vi "SetPressure_v2.vi"(2 "Debug Mode":bool, 3 "Elapsed Time (s)":dbl, 4 "State":enum16{"Edit", "Start", "Run", "End", "Idle"}(ring), 5 "Argument List In":string[](array[string])) -> (0 "Status Out":string, 1 "Argument List Out":string[](array[string]))   [LabVIEW 2011]
panel:
  out "error out":errorcluster
  in  "Dilution factor":dbl min=0.0 max=10.0 format="%.2f"
  in  "Set Point":string(combo)="C"
  in  "P (Torr)":dbl=20.0 format="%.1f"
  in  "Cancel":bool
  in  "OK":bool
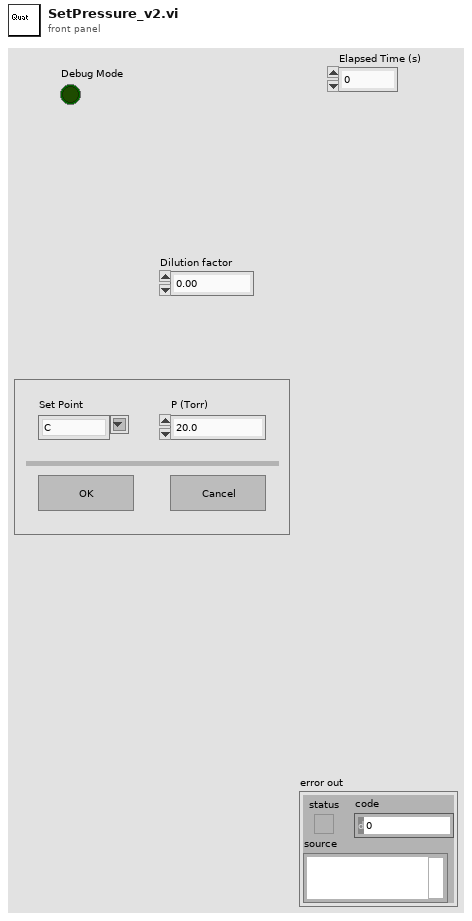
[diagram p1: front panel]
types:
  T1 = enum16{"Discrete", "Continuous", "Instantaneous"}
  T2 = enum32{"Invalid", "Default", "Floating", "Floating/Auto-Hide", "Modal"}
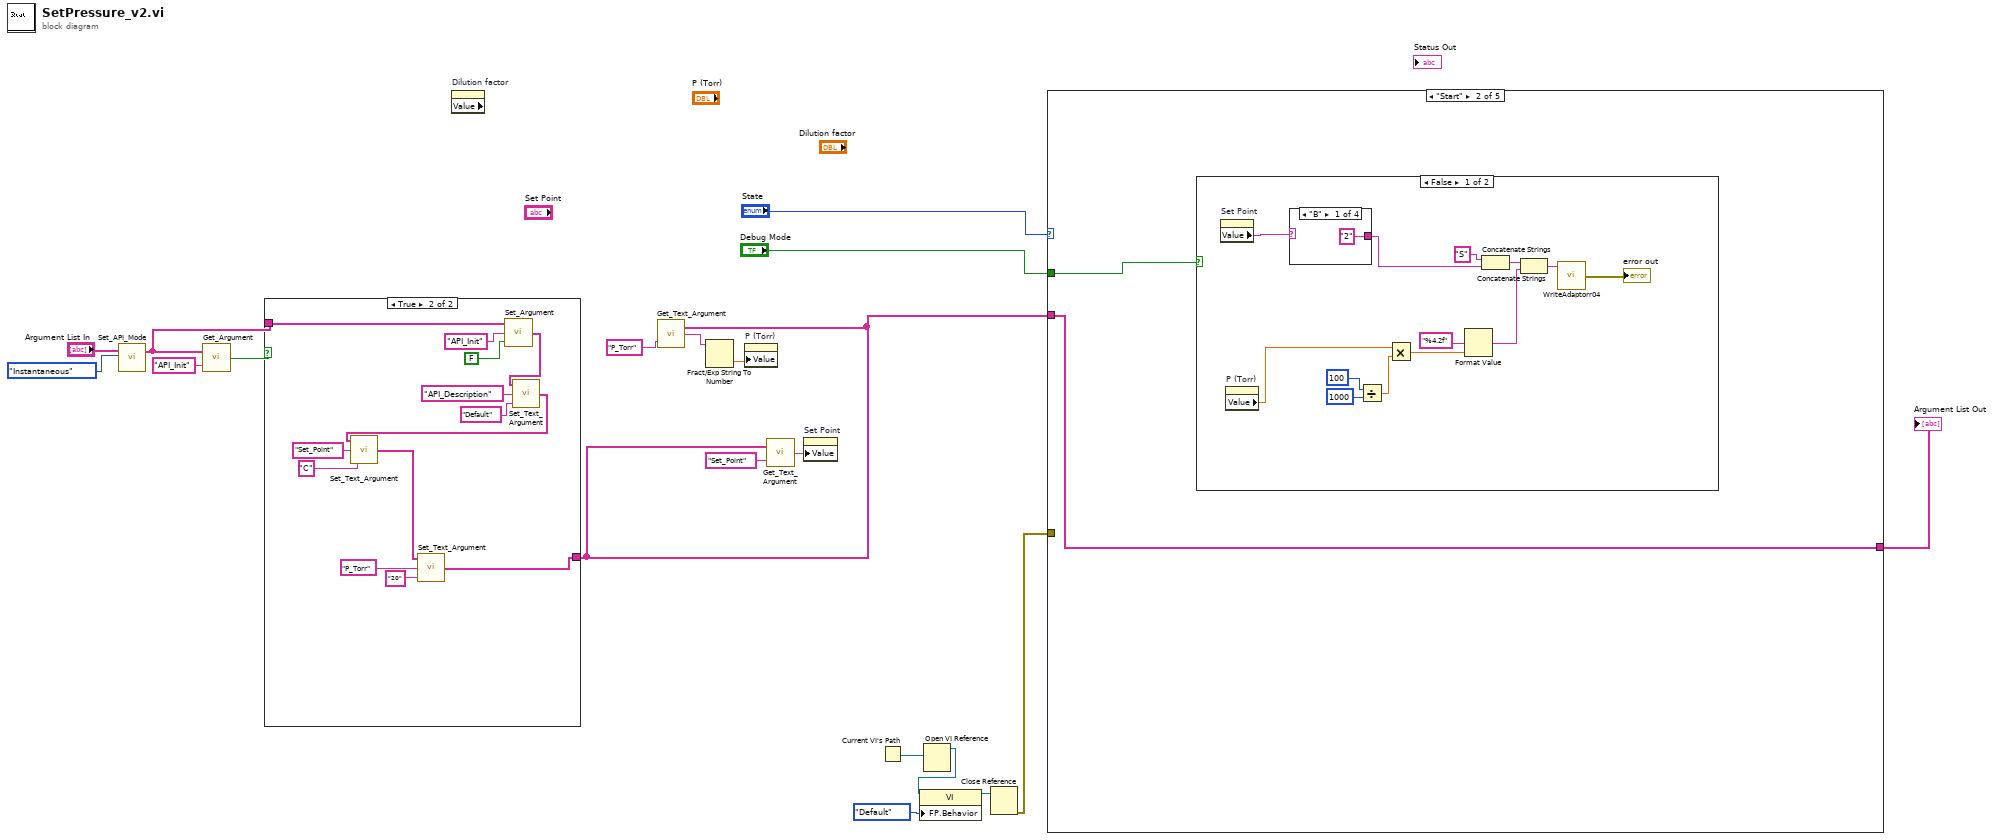
[diagram p0: block diagram]
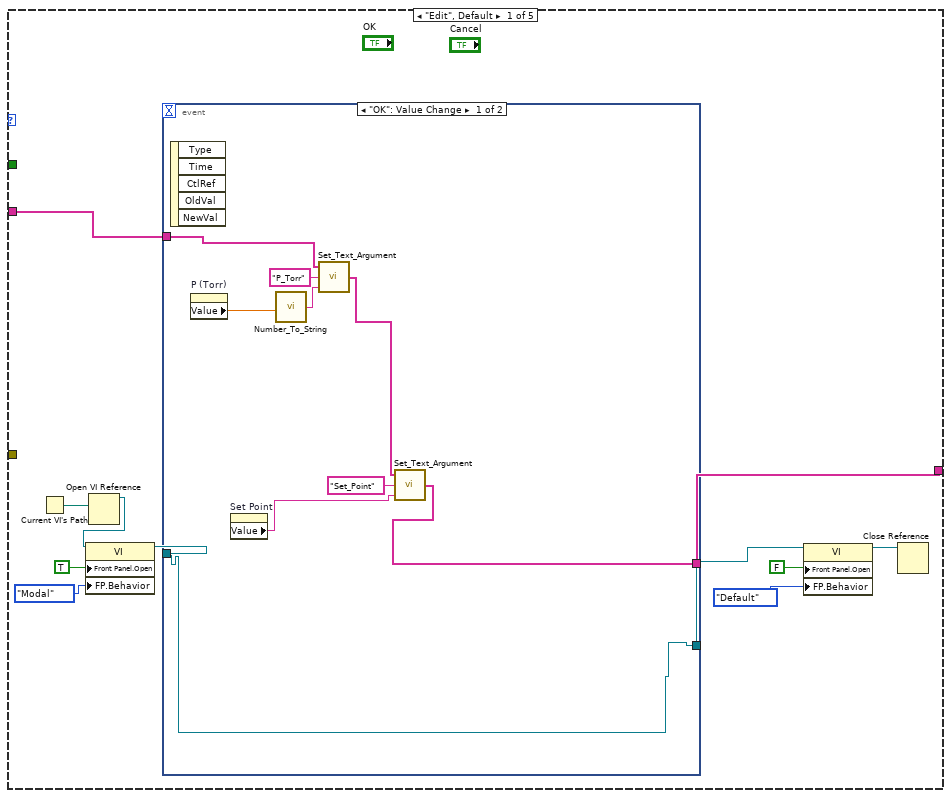
[diagram p3: hidden frame]
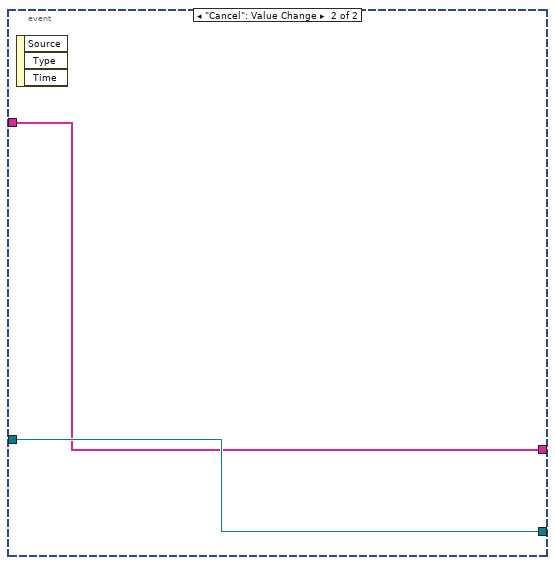
[diagram p4: hidden frame]
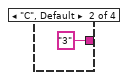
[diagram p5: hidden frame]
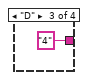
[diagram p6: hidden frame]
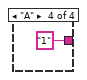
[diagram p7: hidden frame]
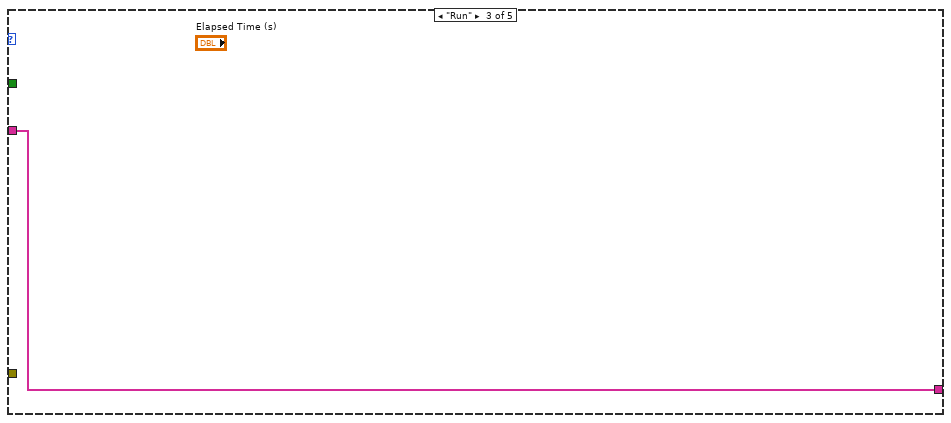
[diagram p9: hidden frame]
diagram:
  n1 = call "Set_API_Mode.vi"("API Mode"=T1."Instantaneous", "Argument List In"="Argument List In") -> ("Argument List Out"=w7:string[])  [unwired: 3 in]
  n2 = call "Get_Argument.vi"("Argument"="API_Init", "Argument List"=w7) -> ("Enabled"=w8:bool)
  n3 = case shown="True" w8 {
    tunnel: w7 -> [w20 w33]
    tunnel: [w20 w23] -> w3
    frame False {
    }
    frame True {
      n4 = call "Set_Argument.vi"("Enable"=FALSE, "Argument"="API_Init", "Argument List In"=w33) -> ("Argument List Out"=w30:string[])
      n5 = call "Set_Text_Argument.vi"("Text"="Default", "Argument"="API_Description", "Argument List In"=w30) -> ("Argument List Out"=w25:string[])
      n6 = call "Set_Text_Argument.vi"("Text"="C", "Argument"="Set_Point", "Argument List In"=w25) -> ("Argument List Out"=w24:string[])
      n7 = call "Set_Text_Argument.vi"("Text"="20", "Argument"="P_Torr", "Argument List In"=w24) -> ("Argument List Out"=w23:string[])
    }
  }
  n8 = property on="Dilution factor" class="DigNum (strict)" props=["Value"]() -> ()  [unwired: 2 in, 3 out]
  n9 = call "Get_Text_Argument.vi"("Argument"="P_Torr", "Argument List"=w3) -> ("Text"=w5:string)
  n10 = Fract/Exp String To Number(string=w5) -> (number=w4:dbl)  [unwired: 4 out]
  n11 = property on="P (Torr)" class="DigNum (strict)"("Value"=w4) -> ()  [unwired: 2 in, 2 out]
  n12 = call "Get_Text_Argument.vi"("Argument"="Set_Point", "Argument List"=w3) -> ("Text"=w1:string)
  n13 = property on="Set Point" class="CmbBox"("Value"=w1) -> ()  [unwired: 2 in, 2 out]
  n14 = Current VI's Path() -> (path=w16:path)
  n15 = Open VI Reference(vi path=w16) -> (vi reference=w15:refnum<vi>)  [unwired: 1 in, 5 out]
  n16 = property class="VI"(reference=w15, "FP.Behavior"=T2."Default" ("Front Panel Window:Behavior")) -> (reference out=w13:refnum<vi>)  [unwired: 1 in, 1 out]
  n17 = Close Reference(reference=w13) -> (error out=w12:errorcluster)  [unwired: 1 in]
  n18 = case shown="\"Start\"" "State" {
    tunnel: [w44 w57 w75 w76 w77] -> w18
    tunnel: w3 -> [w43 w57 w75 w76 w77]
    tunnel: "Debug Mode" -> [_ w56 _ _ _]
    tunnel: w12 -> [_ _ _ _ _]
    frame "Edit", Default {
      n19 = Current VI's Path() -> (path=w38:path)
      n20 = Open VI Reference(vi path=w38) -> (vi reference=w37:refnum<vi>)  [unwired: 1 in, 5 out]
      n21 = property class="VI"(reference=w37, "Front Panel.Open"=TRUE ("Front Panel Window:Open"), "FP.Behavior"=T2."Modal" ("Front Panel Window:Behavior")) -> (reference out=w41:refnum<vi>)  [unwired: 1 in, 1 out]
      n22 = event shown="[0] \"OK\": Value Change" {
        selector: _ -> [_ _]
        dyn-events: _ -> [_ _]
        timeout: _ -> [_ _]
        tunnel: w43 -> [w50 w54]
        tunnel: [w46 w54] -> w44
        tunnel: [w48 w55] -> w40
        tunnel: w41 -> [w48 w55]
        event "OK": Value Change {
          n23 = event-data() -> ()  [unwired: 6 out]
          n24 = property on="P (Torr)" class="DigNum (strict)"() -> ("Value"=w47:dbl)  [unwired: 2 in, 2 out]
          n25 = property on="Set Point" class="CmbBox"() -> ("Value"=w45:string)  [unwired: 2 in, 2 out]
          n26 = call "Number_To_String.vi"("Number"=w47) -> ("String"=w51:string)
          n27 = call "Set_Text_Argument.vi"("Text"=w51, "Argument"="P_Torr", "Argument List In"=w50) -> ("Argument List Out"=w49:string[])
          n28 = call "Set_Text_Argument.vi"("Text"=w45, "Argument"="Set_Point", "Argument List In"=w49) -> ("Argument List Out"=w46:string[])
        }
        event "Cancel": Value Change {
          n29 = event-data() -> ()  [unwired: 4 out]
        }
      }
      n30 = property class="VI"(reference=w40, "Front Panel.Open"=FALSE ("Front Panel Window:Open"), "FP.Behavior"=T2."Default" ("Front Panel Window:Behavior")) -> (reference out=w34:refnum<vi>)  [unwired: 1 in, 1 out]
      n31 = Close Reference(reference=w34) -> ()  [unwired: 1 in, 1 out]
    }
    frame "Start" {
      n32 = case shown="False" w56 {
        frame False {
          n33 = property on="Set Point" class="CmbBox"() -> ("Value"=w60:string)  [unwired: 2 in, 2 out]
          n34 = property on="P (Torr)" class="DigNum (strict)"() -> ("Value"=w58:dbl)  [unwired: 2 in, 2 out]
          n35 = case shown="\"B\"" w60 {
            tunnel: ["2" "3" "4" "1"] -> w59
            frame "B" {
            }
            frame "C", Default {
            }
            frame "D" {
            }
            frame "A" {
            }
          }
          n36 = Divide(x=100, y=1000) -> (x/y=w66:dbl)
          n37 = Multiply(x=w58, y=w66) -> (x*y=w69:dbl)
          n38 = Format Value(format string="%4.2f", value (0)=w69) -> (output string=w70:string)  [unwired: 1 in]
          n39 = Concatenate Strings("S", w59) -> (w62:string)
          n40 = Concatenate Strings(w62, w70) -> (w67:string)
          n41 = call "WriteAdaptorr04.vi"("string to write"=w67) -> ("error out"=→"error out":errorcluster)  [unwired: 2 in]
        }
        frame True {
        }
      }
    }
    frame "Run" {
    }
    frame "End" {
    }
    frame "Idle" {
    }
  }
  "Argument List Out" <- w18
